vi "Start Tx.vi"(6 "error in (no error)":errorcluster, 8 "TX PARAMETER PANEL":T1={"Chain Mask"=0, "CF(MHz)"=2412, "CF2(MHz)"=0, "Data Rate"=0, "TX Power, dB"=0.0, "Packet Length"=1500, "Packet Count"=0, "LDPC?"=FALSE, "DPD?"=FALSE} {"Chain Mask" items=["0x1 : ch0"=1, "0x2 : ch1"=2, "0x4 : ch2"=4, "0x8 : ch3"=8, "0x3 : ch0, ch1"=3, "0x7 : ch0, ch1, ch2"=7, "0x15 : ch0, ch1, ch2, ch3"=15, "0x5 : ch0, ch2"=5, "0x10 : ch1, ch3"=10, "0x9 : ch1, ch3"=9, "0x12 : ch2, ch4"=12]; "Data Rate" items=["RATE_1Mbps"=0, "RATE_2Mbps"=1, "RATE_5_5Mbps"=2, "RATE_11Mbps"=3, "RATE_6Mbps"=4, "RATE_9Mbps"=5, "RATE_12Mbps"=6, "RATE_18Mbps"=7, "RATE_24Mbps"=8, "RATE_36Mbps"=9, "RATE_48Mbps"=10, "RATE_54Mbps"=11, "RATE_MCS_0_20"=12, "RATE_MCS_1_20"=13, "RATE_MCS_2_20"=14, "RATE_MCS_3_20"=15, "RATE_MCS_4_20"=16, "RATE_MCS_5_20"=17, "RATE_MCS_6_20"=18, "RATE_MCS_7_20"=19, "RATE_MCS_0_40"=20, "RATE_MCS_1_40"=21, "RATE_MCS_2_40"=22, "RATE_MCS_3_40"=23, "RATE_MCS_4_40"=24, "RATE_MCS_5_40"=25, "RATE_MCS_6_40"=26, "RATE_MCS_7_40"=27, "RATE_AC_MCS_0_20"=28, "RATE_AC_MCS_1_20"=29, "RATE_AC_MCS_2_20"=30, "RATE_AC_MCS_3_20"=31, "RATE_AC_MCS_4_20"=32, "RATE_AC_MCS_5_20"=33, "RATE_AC_MCS_6_20"=34, "RATE_AC_MCS_7_20"=35, "RATE_AC_MCS_8_20"=36, "RATE_AC_MCS_9_20"=37, "RATE_AC_MCS_0_40"=38, "RATE_AC_MCS_1_40"=39, "RATE_AC_MCS_2_40"=40, "RATE_AC_MCS_3_40"=41, "RATE_AC_MCS_4_40"=42, "RATE_AC_MCS_5_40"=43, "RATE_AC_MCS_6_40"=44, "RATE_AC_MCS_7_40"=45, "RATE_AC_MCS_8_40"=46, "RATE_AC_MCS_9_40"=47, "RATE_AC_MCS_0_80"=48, "RATE_AC_MCS_1_80"=49, "RATE_AC_MCS_2_80"=50, "RATE_AC_MCS_3_80"=51, "RATE_AC_MCS_4_80"=52, "RATE_AC_MCS_5_80"=53, "RATE_AC_MCS_6_80"=54, "RATE_AC_MCS_7_80"=55, "RATE_AC_MCS_8_80"=56, "RATE_AC_MCS_9_80"=57, "RATE_MCS_8_20"=58, "RATE_MCS_9_20"=59, "RATE_MCS_10_20"=60, "RATE_MCS_11_20"=61, "RATE_MCS_12_20"=62, "RATE_MCS_13_20"=63, "RATE_MCS_14_20"=64, "RATE_MCS_15_20"=65, "RATE_MCS_8_40"=66, "RATE_MCS_9_40"=67, "RATE_MCS_10_40"=68, "RATE_MCS_11_40"=69, "RATE_MCS_12_40"=70, "RATE_MCS_13_40"=71, "RATE_MCS_14_40"=72, "RATE_MCS_15_40"=73, "RATE_AC_MCS_10_20"=74, "RATE_AC_MCS_11_20"=75, "RATE_AC_MCS_12_20"=76, "RATE_AC_MCS_13_20"=77, "RATE_AC_MCS_14_20"=78, "RATE_AC_MCS_15_20"=79, "RATE_AC_MCS_16_20"=80, "RATE_AC_MCS_17_20"=81, "RATE_AC_MCS_18_20"=82, "RATE_AC_MCS_19_20"=83, "RATE_AC_MCS_10_40"=84, "RATE_AC_MCS_11_40"=85, "RATE_AC_MCS_12_40"=86, "RATE_AC_MCS_13_40"=87, "RATE_AC_MCS_14_40"=88, "RATE_AC_MCS_15_40"=89, "RATE_AC_MCS_16_40"=90, "RATE_AC_MCS_17_40"=91, "RATE_AC_MCS_18_40"=92, "RATE_AC_MCS_19_40"=93, "RATE_AC_MCS_10_80"=94, "RATE_AC_MCS_11_80"=95, "RATE_AC_MCS_12_80"=96, "RATE_AC_MCS_13_80"=97, "RATE_AC_MCS_14_80"=98, "RATE_AC_MCS_15_80"=99, "RATE_AC_MCS_16_80"=100, "RATE_AC_MCS_17_80"=101, "RATE_AC_MCS_18_80"=102, "RATE_AC_MCS_19_80"=103, "RATE_MCS_16_20"=104, "RATE_MCS_17_20"=105, "RATE_MCS_18_20"=106, "RATE_MCS_19_20"=107, "RATE_MCS_20_20"=108, "RATE_MCS_21_20"=109, "RATE_MCS_22_20"=110, "RATE_MCS_23_20"=111, "RATE_MCS_16_40"=112, "RATE_MCS_17_40"=113, "RATE_MCS_18_40"=114, "RATE_MCS_19_40"=115, "RATE_MCS_20_40"=116, "RATE_MCS_21_40"=117, "RATE_MCS_22_40"=118, "RATE_MCS_23_40"=119, "RATE_AC_MCS_20_20"=120, "RATE_AC_MCS_21_20"=121, "RATE_AC_MCS_22_20"=122, "RATE_AC_MCS_23_20"=123, "RATE_AC_MCS_24_20"=124, "RATE_AC_MCS_25_20"=125, "RATE_AC_MCS_26_20"=126, "RATE_AC_MCS_27_20"=127, "RATE_AC_MCS_28_20"=128, "RATE_AC_MCS_29_20"=129, "RATE_AC_MCS_20_40"=130, "RATE_AC_MCS_21_40"=131, "RATE_AC_MCS_22_40"=132, "RATE_AC_MCS_23_40"=133, "RATE_AC_MCS_24_40"=134, "RATE_AC_MCS_25_40"=135, "RATE_AC_MCS_26_40"=136, "RATE_AC_MCS_27_40"=137, "RATE_AC_MCS_28_40"=138, "RATE_AC_MCS_29_40"=139, "RATE_AC_MCS_20_80"=140, "RATE_AC_MCS_21_80"=141, "RATE_AC_MCS_22_80"=142, "RATE_AC_MCS_23_80"=143, "RATE_AC_MCS_24_80"=144, "RATE_AC_MCS_25_80"=145, "RATE_AC_MCS_26_80"=146, "RATE_AC_MCS_27_80"=147, "RATE_AC_MCS_28_80"=148, "RATE_AC_MCS_29_80"=149, "RATE_AC_MCS_30_20"=150, "RATE_AC_MCS_31_20"=151, "RATE_AC_MCS_32_20"=152, "RATE_AC_MCS_33_20"=153, "RATE_AC_MCS_34_20"=154, "RATE_AC_MCS_35_20"=155, "RATE_AC_MCS_36_20"=156, "RATE_AC_MCS_37_20"=157, "RATE_AC_MCS_38_20"=158, "RATE_AC_MCS_39_20"=159, "RATE_AC_MCS_30_40"=160, "RATE_AC_MCS_31_40"=161, "RATE_AC_MCS_32_40"=162, "RATE_AC_MCS_33_40"=163, "RATE_AC_MCS_34_40"=164, "RATE_AC_MCS_35_40"=165, "RATE_AC_MCS_36_40"=166, "RATE_AC_MCS_37_40"=167, "RATE_AC_MCS_38_40"=168, "RATE_AC_MCS_39_40"=169, "RATE_AC_MCS_30_80"=170, "RATE_AC_MCS_31_80"=171, "RATE_AC_MCS_32_80"=172, "RATE_AC_MCS_33_80"=173, "RATE_AC_MCS_34_80"=174, "RATE_AC_MCS_35_80"=175, "RATE_AC_MCS_36_80"=176, "RATE_AC_MCS_37_80"=177, "RATE_AC_MCS_38_80"=178, "RATE_AC_MCS_39_80"=179, "RATE_AC_MCS_0_160"=180, "RATE_AC_MCS_1_160"=181, "RATE_AC_MCS_2_160"=182, "RATE_AC_MCS_3_160"=183, "RATE_AC_MCS_4_160"=184, "RATE_AC_MCS_5_160"=185, "RATE_AC_MCS_6_160"=186, "RATE_AC_MCS_7_160"=187, "RATE_AC_MCS_8_160"=188, "RATE_AC_MCS_9_160"=189, "RATE_AC_MCS_10_160"=190, "RATE_AC_MCS_11_160"=191, "RATE_AC_MCS_12_160"=192, "RATE_AC_MCS_13_160"=193, "RATE_AC_MCS_14_160"=194, "RATE_AC_MCS_15_160"=195, "RATE_AC_MCS_16_160"=196, "RATE_AC_MCS_17_160"=197, "RATE_AC_MCS_18_160"=198, "RATE_AC_MCS_19_160"=199, "RATE_MCS_24_20"=220, "RATE_MCS_25_20"=221, "RATE_MCS_26_20"=222, "RATE_MCS_27_20"=223, "RATE_MCS_28_20"=224, "RATE_MCS_29_20"=225, "RATE_MCS_30_20"=226, "RATE_MCS_31_20"=227, "RATE_MCS_24_40"=228, "RATE_MCS_25_40"=229, "RATE_MCS_26_40"=230, "RATE_MCS_27_40"=231, "RATE_MCS_28_40"=232, "RATE_MCS_29_40"=233, "RATE_MCS_30_40"=234, "RATE_MCS_31_40"=235, "RATE_P_1p5Mbps_5"=1004, "RATE_P_2Mbps_5"=1005, "RATE_P_3Mbps_5"=1006, "RATE_P_4p5Mbps_5"=1007, "RATE_P_6Mbps_5"=1008, "RATE_P_9Mbps_5"=1009, "RATE_P_12Mbps_5"=1010, "RATE_P_13p5Mbps_5"=1011, "RATE_P_3Mbps_10"=1104, "RATE_P_4p5Mbps_10"=1105, "RATE_P_6Mbps_10"=1106, "RATE_P_9Mbps_10"=1107, "RATE_P_12Mbps_10"=1108, "RATE_P_18Mbps_10"=1109, "RATE_P_24Mbps_10"=1110, "RATE_P_27Mbps_10"=1111, "RATE_P_6Mbps_20"=1204, "RATE_P_9Mbps_20"=1205, "RATE_P_12Mbps_20"=1206, "RATE_P_18Mbps_20"=1207, "RATE_P_24Mbps_20"=1208, "RATE_P_36Mbps_20"=1209, "RATE_P_48Mbps_20"=1210, "RATE_P_54Mbps_20"=1211]}, 9 "_hResourceContext":u32) -> (0 "error out":errorcluster, 2 "function return":bool, 3 "_hResourceContext out":u32)   [LabVIEW 2013, in "QCAWLAN_DLL.lvlib"]
doc: "QCA_DLL_Export bool StartTx(HANDLE _hResourceContext, int channel, int wlanMode, int rateBitIndex0, int tpcm, int txMode, int txChain0, int txPower0, int gainIdx, int dacGain, int paConfig, int pktLen0, int shortGuard, bool ldpcRate, bool STBCmode, int agg, bool dpdMode, int numPackets, int broadcast, int AIFSN, int channel2, int cbState);"
uses:
  QCAWLAN_DLL.lvlib
  TypeDef/TX PARAMETER PANEL.ctl
  TypeDef/CHAIN_MASK.ctl
  TypeDef/TX DATA RATE.ctl
  TypeDef/TX SETUP PARAMETER.ctl
  TypeDef/TX POWER CONTROL.ctl
  QCAWLAN_DLL.dll
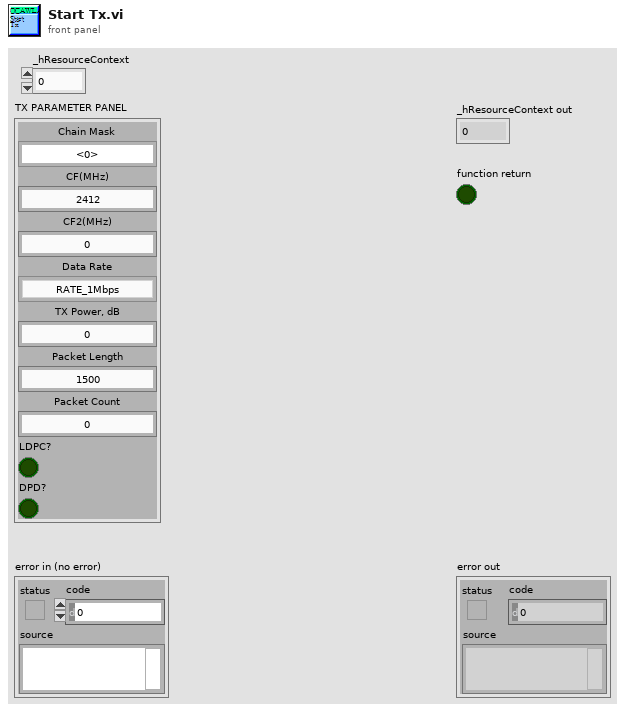
[diagram p1: front panel]
types:
  T1 = typedef "TX PARAMETER PANEL.ctl" = cluster{"Chain Mask":T2, "CF(MHz)":u32, "CF2(MHz)":u32, "Data Rate":T3, "TX Power, dB":dbl, "Packet Length":u32, "Packet Count":i32, "LDPC?":bool, "DPD?":bool}
  T2 = typedef "CHAIN_MASK.ctl" = u16
  T3 = typedef "TX DATA RATE.ctl" = u16
  T4 = typedef "TX POWER CONTROL.ctl" = enum16{"ForcedGain", "OpenLoopSearch", "TxPowerAuto", "TxPowerForce_CLPC", "TxPowerForce_SCPC", "TxPowerForce_OLPC", "ForcedDesiredGain", "ForcedGLUTIndex"}
  T5 = typedef "TX SETUP PARAMETER.ctl" = cluster{"channel":i32, "wlanMode":i32, "rateBitIndex0":i32, "tpcm":i32, "txMode":i32, "txChain0":i32, "txPower0":i32, "gainIdx":i32, "dacGain":i32, "paConfig":i32, "pktLen0":i32, "shortGuard":i32, "ldpcRate":bool, "STBCmode":bool, "agg":i32, "dpdMode":bool, "numPackets":i32, "broadcast":i32, "AIFSN":i32, "channel2":i32, "cbstate":i32}
  T6 = typedef "CHANNEL BONDING STATE.ctl" = u16
  T7 = typedef "WLAN MODE.ctl" = u16
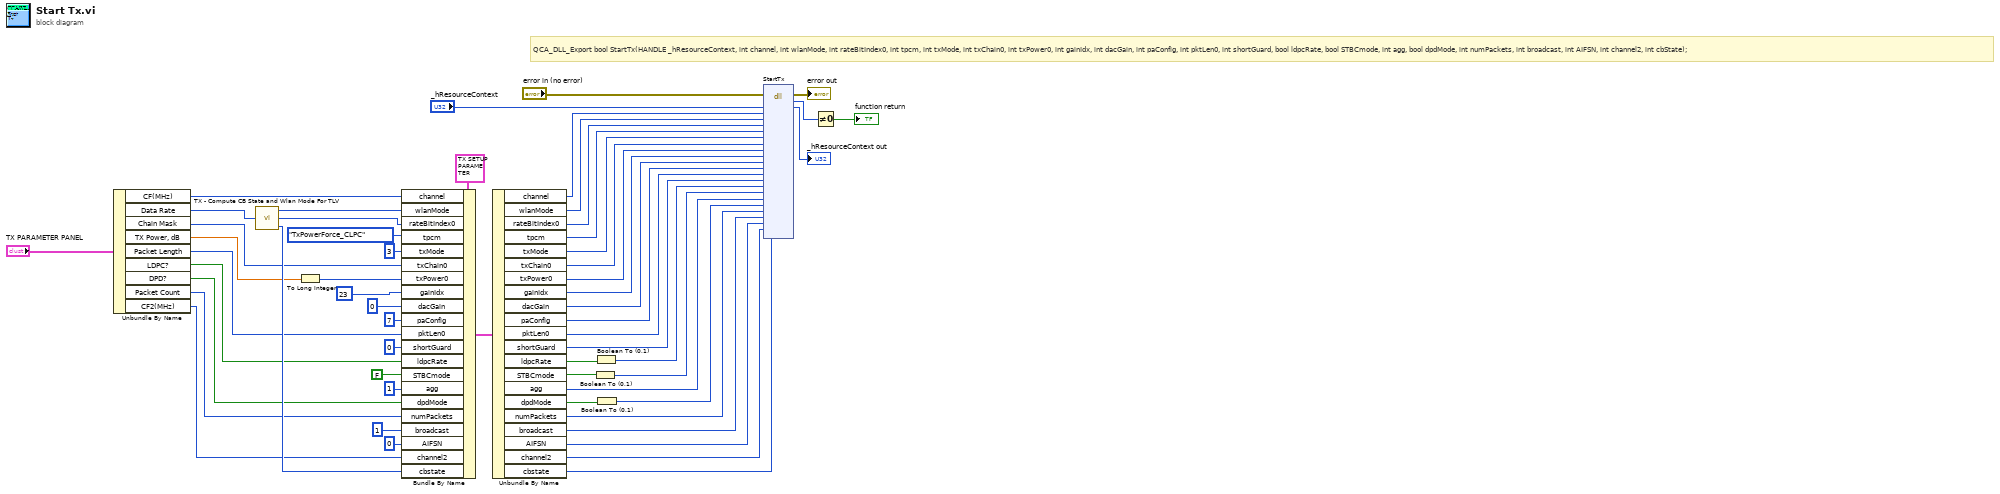
[diagram p0: block diagram]
diagram:
  # "QCA_DLL_Export bool StartTx(HANDLE _hResourceContext, int channel, int wlanMode, int rateBitIndex0, int tpcm, int txMode, int txChain0, int txPower0, int gainIdx, int dacGain, int paConfig, int pktLen0, int shortGuard, bool ldpcRate, bool STBCmode, int agg, bool dpdMode, int numPackets, int broadcast, int AIFSN, int channel2, int cbState);"
  n1 = Unbundle By Name("TX PARAMETER PANEL") -> ("CF(MHz)"=w45:u32, "Data Rate"=w46:T3, "Chain Mask"=w42:T2, "TX Power, dB"=w41:dbl, "Packet Length"=w37:u32, "LDPC?"=w1:bool, "DPD?"=w36:bool, "Packet Count"=w32:i32, "CF2(MHz)"=w31:u32)
  n2 = call "TX - Compute CB State and Wlan Mode For TLV.vi"("TX Data Rate"=w46) -> ("ChannelBondingState"=w47:T6, "TLV Rate"=w48:i32, "WLAN Mode"=w49:T7)  [unwired: 2 in]
  n3 = To Long Integer(number=w41) -> (32bit integer=w2:i32)
  n4 = Bundle By Name(cluster=T5 {"channel"=0, "wlanMode"=0, "rateBitIndex0"=0, "tpcm"=0, "txMode"=0, "txChain0"=0, "txPower0"=0, "gainIdx"=0, "dacGain"=0, "paConfig"=0, "pktLen0"=0, "shortGuard"=0, "ldpcRate"=FALSE, "STBCmode"=FALSE, "agg"=0, "dpdMode"=FALSE, "numPackets"=0, "broadcast"=0, "AIFSN"=0, "channel2"=0, "cbstate"=0} ("Tx Parameters"), "channel"=w45, "wlanMode"=w49, "rateBitIndex0"=w48, "tpcm"=TX_POWER_CONTROL."TxPowerForce_CLPC" ("Tx Power Control"), "txMode"=3, "txChain0"=w42, "txPower0"=w2, "gainIdx"=23, "dacGain"=0, "paConfig"=7, "pktLen0"=w37, "shortGuard"=0, "ldpcRate"=w1, "STBCmode"=FALSE, "agg"=1, "dpdMode"=w36, "numPackets"=w32, "broadcast"=1, "AIFSN"=0, "channel2"=w31, "cbstate"=w47) -> (w27:T5)
  n5 = Unbundle By Name(w27) -> ("channel"=w26:i32, "wlanMode"=w25:i32, "rateBitIndex0"=w24:i32, "tpcm"=w23:i32, "txMode"=w22:i32, "txChain0"=w21:i32, "txPower0"=w20:i32, "gainIdx"=w19:i32, "dacGain"=w18:i32, "paConfig"=w17:i32, "pktLen0"=w16:i32, "shortGuard"=w15:i32, "ldpcRate"=w14:bool, "STBCmode"=w12:bool, "agg"=w10:i32, "dpdMode"=w9:bool, "numPackets"=w7:i32, "broadcast"=w6:i32, "AIFSN"=w5:i32, "channel2"=w4:i32, "cbstate"=w3:i32)
  n6 = Boolean To (0,1)(Boolean=w12) -> (0, 1=w11:i16)
  n7 = Boolean To (0,1)(Boolean=w14) -> (0, 1=w13:i16)
  n8 = Boolean To (0,1)(Boolean=w9) -> (0, 1=w8:i16)
  n9 = dll-call lib="C:/Connectivity Client - MIMO/PlugIn/QCAWLAN_DLL.*" fn="StartTx"(error in="error in (no error)", "_hResourceContext"="_hResourceContext", "channel"=w26, "wlanMode"=w25, "rateBitIndex0"=w24, "tpcm"=w23, "txMode"=w22, "txChain0"=w21, "txPower0"=w20, "gainIdx"=w19, "dacGain"=w18, "paConfig"=w17, "pktLen0"=w16, "shortGuard"=w15, "ldpcRate"=w13, "STBCmode"=w11, "agg"=w10, "dpdMode"=w8, "numPackets"=w7, "broadcast"=w6, "AIFSN"=w5, "channel2"=w4, "cbState"=w3) -> (error out=→"error out":errorcluster, w55:u8, "_hResourceContext"=→"_hResourceContext out":u32)  [unwired: 23 in, 1 out]
  n10 = Not Equal To 0?(x=w55) -> (x != 0?=→"function return":bool)
